vi "ThresholdLevelFinderNEW.vi"(5 "correction":i32, 6 "Initial Threshold":i32=500, 7 "Channel":u32, 8 "error in (no error)":errorcluster, 9 "id_in":i32, 10 "connection ID":refnum<k5>, 11 "VISA resource name":refnum<visa-resource-name>="AgilentOsciloscope") -> (0 "error out":errorcluster, 1 "id_out":i32, 2 "connection ID out":refnum<k5>, 3 "VISA resource name out":refnum<visa-resource-name>="AgilentOsciloscope", 4 "threshold out":i32=511)   [LabVIEW 2012]
uses:
  Sum_Abrilader/L0_Sum_Adder Folder/C/Program Files/National Instruments/LabVIEW 2012/instr.lib/Agilent 8000 Series/Public/Data/Low Level/Fetch Measurement (More).vi
  <instrlib>/Agilent 8000 Series/Agilent 8000 Series.lvlib
panel:
  in  "increment":i32=2
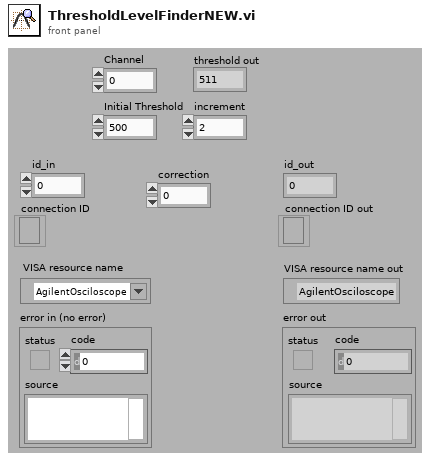
[diagram p1: front panel]
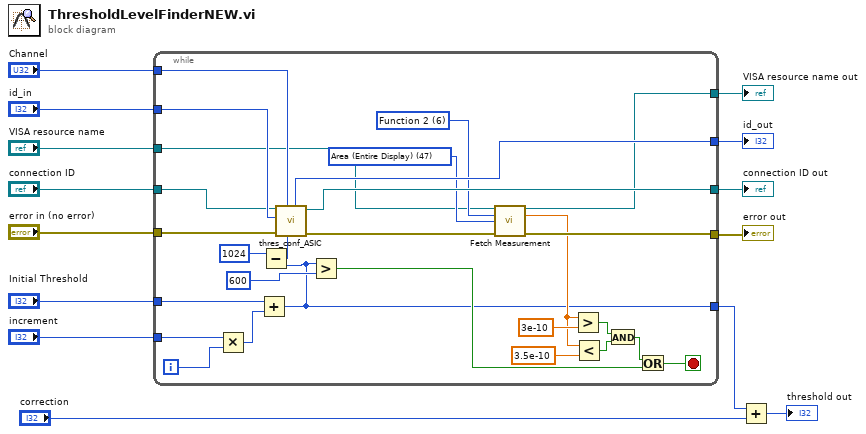
[diagram p0: block diagram]
diagram:
  n1 = while {
    tunnel: "VISA resource name" -> [w28]
    tunnel: [w27] -> w13
    tunnel: "connection ID" -> [w32]
    tunnel: [w42] -> w11
    tunnel: "error in (no error)" -> [w31]
    tunnel: "id_in" -> [w38]
    tunnel: [w37] -> w8
    tunnel: "Channel" -> [w36]
    tunnel: [w17] -> w2
    tunnel: "Initial Threshold" -> [w35]
    tunnel: "increment" -> [w34]
    tunnel: [w26] -> w4
    i -> [w40]
    stop <- w25 stop-if-true
    w30 = 47 items=["Rise Time", "Fall Time", "Frequency", "Period", "Voltage RMS(AC)", "Voltage RMS(DC)", "Voltage RMS (AC,cycle)", "Voltage RMS (DC,cycle)", "Voltage Max", "Voltage Min", "Voltage Middle", "Voltage Vpp", "Voltage High", "Voltage Low", "Voltage Average", "Voltage Average (cycle)", "Width Negative", "Width Positive", "Duty Cycle Positive", "Amplitude", "Overshoot", "Preshoot", "Voltage Base", "Voltage Upper", "Time Max", "Time Min", "Color Grade Crossing", "Color Grade Eye Width", "Color Grade Eye Height", "Color Grade Eye Q-Factory", "Color Grade Eye Duty Cycle Distortion(Percent)", "Color Grade Eye Duty Cycle Distortion(Time)", "Color Grade Eye Jitter(PP)", "Color Grade Eye Width(RMS)", "Cycle-cycle Duty Jitter(Rising)", "Cycle-cycle Duty Jitter(Falling)", "Cycle-cycle Jitter(Rising)", "Cycle-cycle Jitter(Falling)", "Cycle-cycle - Width", "Cycle-cycle + Width", "Date Rate", "Unit Interval", "FFT Delta Frequency", "FFT Delta Magnitude", "FFT Frequency", "FFT Magnitude", "Slew Rate", "Area (Entire Display)", "Area(Single Cycle)", "Duty Cycle (Rising)", "Duty Cycle (Falling)"] ("Measurement Function (0: Rise Time)")
    w29 = 6 items=["Channel 1"=1, "Channel 2"=2, "Channel 3"=3, "Channel 4"=4, "Function 1"=5, "Function 2"=6, "Function 3"=7, "Function 4"=8, "Memory 1"=9, "Memory 2"=10, "Memory 3"=11, "Memory 4"=12] ("Channel (1: Channel 1)")
    n2 = Multiply(x=w34, y=w40) -> (x*y=w39:i32)
    n3 = Add(x=w35, y=w39) -> (x+y=w17:i32)
    n4 = Subtract(x=1024, y=w17) -> (x-y=w16:i32)
    n5 = call "thres_conf_ASIC.vi"("threshold"=w16, "Ring"=w36, "error out 3"=w31, "Id in"=w38, "connection ID"=w32) -> ("error out 2"=w18:errorcluster, "connection ID out"=w42:refnum<k5>, "Id out"=w37:i32)  [unwired: 3 in, 1 out]
    n6 = Greater?(x=w17, y=600) -> (0:w23:bool)
    n7 = call-poly "Fetch Measurement.vi"("VISA resource name"=w28, "Channel (1: Channel 1)"=w29, "Measurement Function (0: Rise Time)"=w30, "error in (no error)"=w18) -> ("VISA resource name out"=w27:refnum<visa-resource-name>, "Measurement"=w22:dbl, "error out"=w26:errorcluster)  [unwired: 9 in]
    n8 = Greater?(x=w22, y=3e-10) -> (0:w24:bool)
    n9 = Less?(x=w22, y=3.5e-10) -> (x < y?=w21:bool)
    n10 = And(x=w24, y=w21) -> (x .and. y?=w19:bool)
    n11 = Or(x=w19, y=w23) -> (x .or. y?=w25:bool)
  }
  "VISA resource name out" <- w13
  "error out" <- w4
  "connection ID out" <- w11
  "id_out" <- w8
  n12 = Add(x=w2, y="correction") -> (x+y=→"threshold out":i32)
